vi "2D String.vi"(7 "key description":string, 8 "sections":string[](array[string]), 9 "string":string[][](array[string]), 11 "info data":string) -> (0 "sections out":string[](array[string]), 3 "info data out":string)   [LabVIEW 2013, in "infolib.lvlib"]
doc: "Add a new string table to Info Data string. If section exists in Info Data string, inserts key into this section."
uses:
  infolib.lvlib
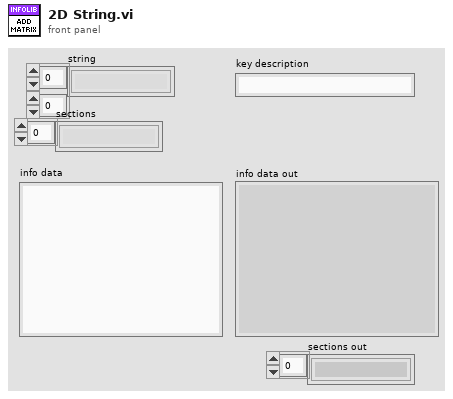
[diagram p1: front panel]
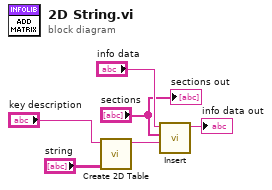
[diagram p0: block diagram]
diagram:
  n1 = call "Create 2D Table.vi"("formatted values"="string", "table name"="key description") -> ("table"=w2:string)  [unwired: 9 in]
  n2 = call "Insert.vi"("insert"=w2, "sections"="sections", "info data"="info data") -> ("info data out"=→"info data out":string)  [unwired: 8 in]
  "sections out" <- "sections"
